vi "User selection GUI.vi"(11 "error in (no error)":errorcluster) -> (8 "OK":bool, 15 "error out":errorcluster)   [LabVIEW 2011]
uses:
  Application Structure/User Control/Super User bool indikator.ctl
  Application Structure/User Control/User Indikator.ctl
  emi Lib/Basic/0 - General/App/Version/Private/_emi_Version Holder.vi
panel:
  in  "User name":string
  in  "Help":bool
  in  "Cancel":bool
  in  "OK btn":bool
  # "Select user name and level"
  # "Tab header s can be changed as wanted\n\nCustom can be used for completly ccutom behavior,\nmust then highjack  an other hidden page, for settings"
  # "Add custom behavior taht cvan not be replicated by a simple cluster with valisdity checking"
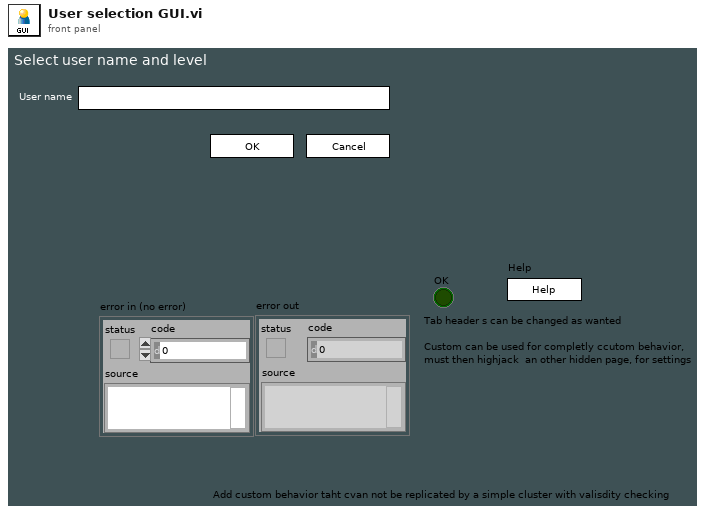
[diagram p1: front panel]
types:
  T1 = enum16{"GET", "SET", "Get from Ini", "Put in Ini"}
  T2 = typedef "User Indikator.ctl" = cluster{"User Name":string, "Super User":T3}
  T3 = typedef "Super User bool indikator.ctl" = bool
  T4 = typedef "emi_Version Info.ctl" = cluster{"Name":string, "Major":i16, "Minor":i16, "Fix":i16, "Build":i32, "Type":enum16{"Alfa", "Beta", "Stable"}, "Dev":bool, "Version Name":string, "Date":timestamp}
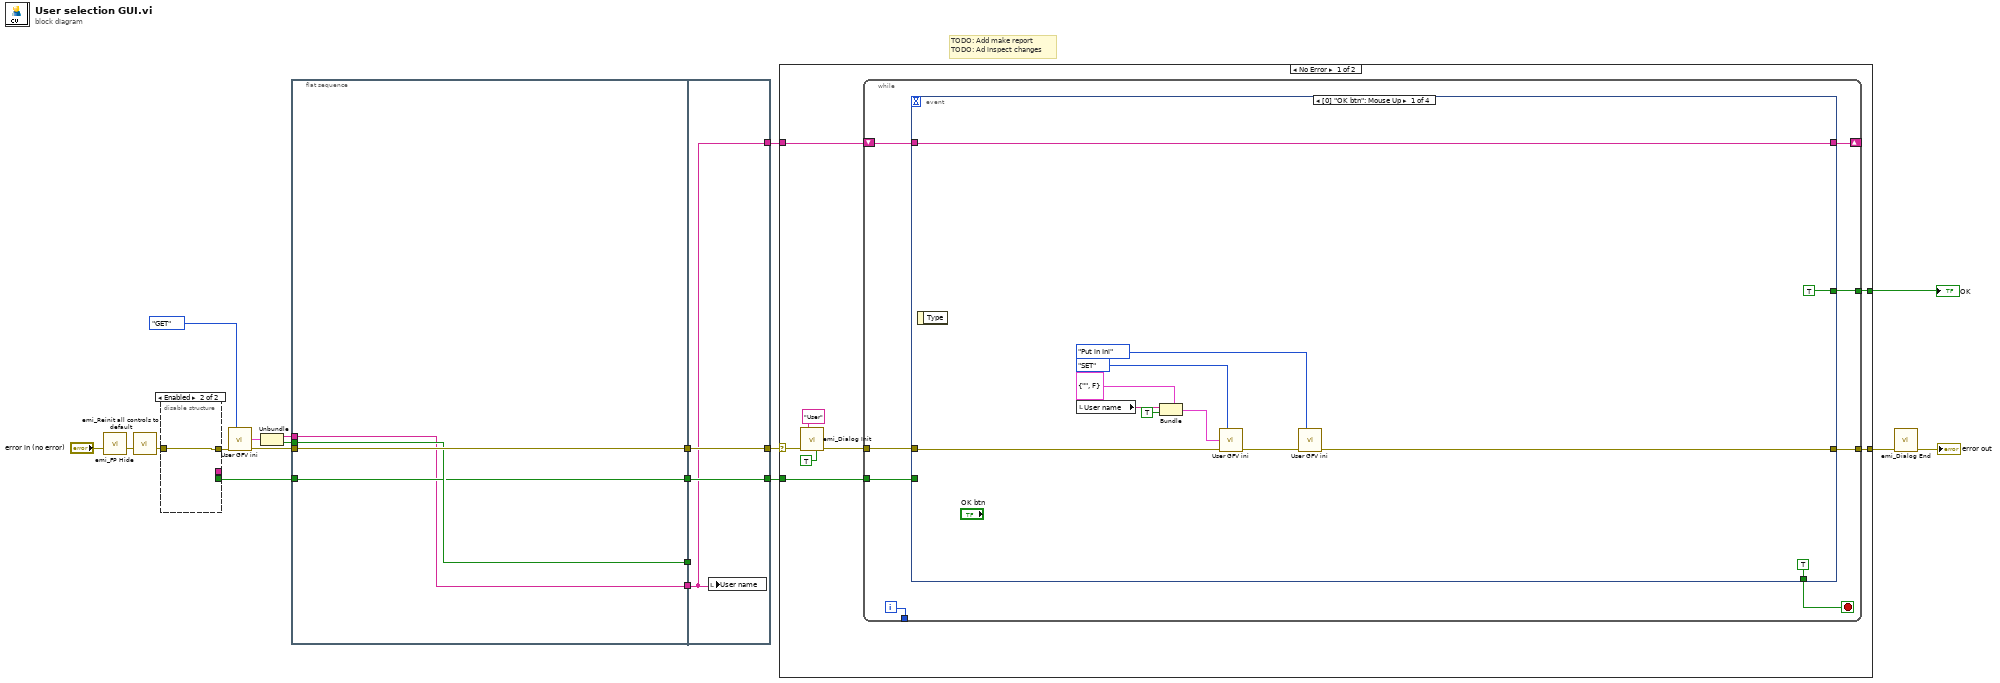
[diagram p0: block diagram]
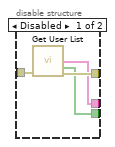
[diagram p2: hidden frame]
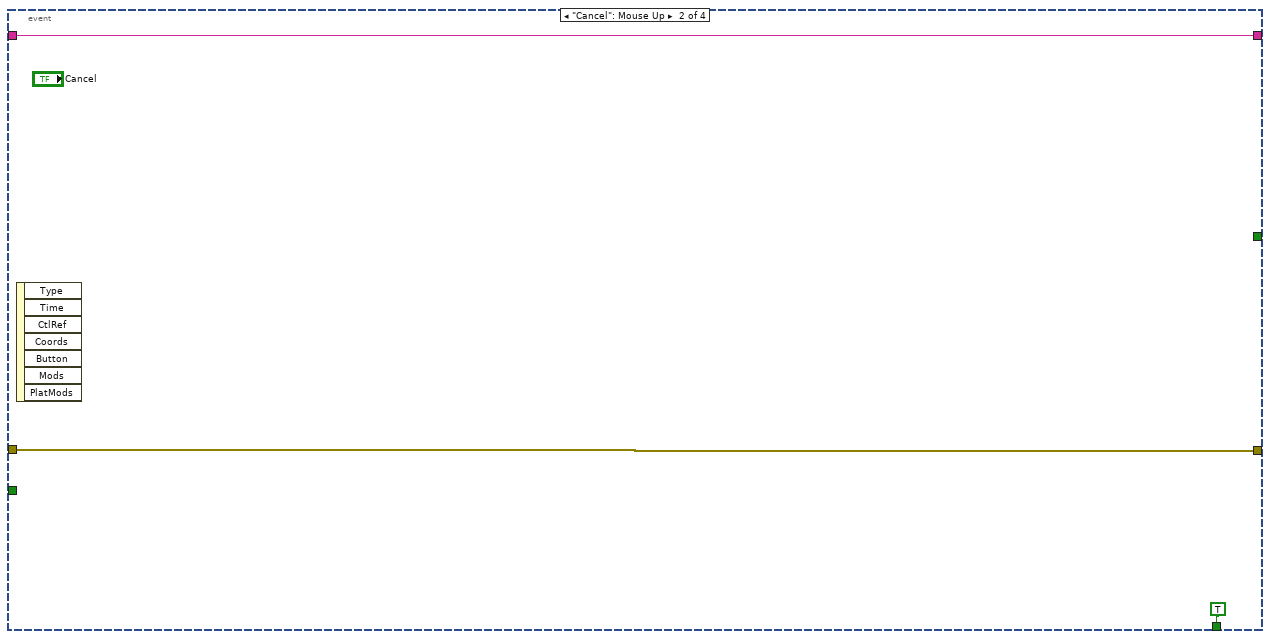
[diagram p3: hidden frame]
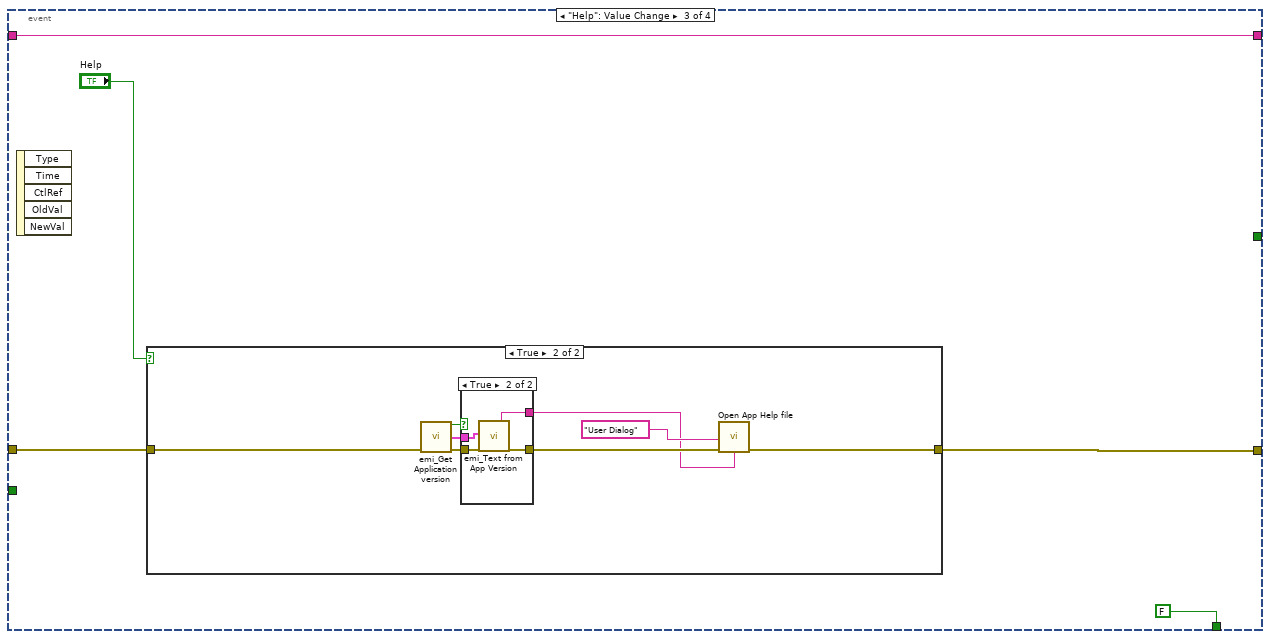
[diagram p4: hidden frame]
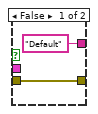
[diagram p6: hidden frame]
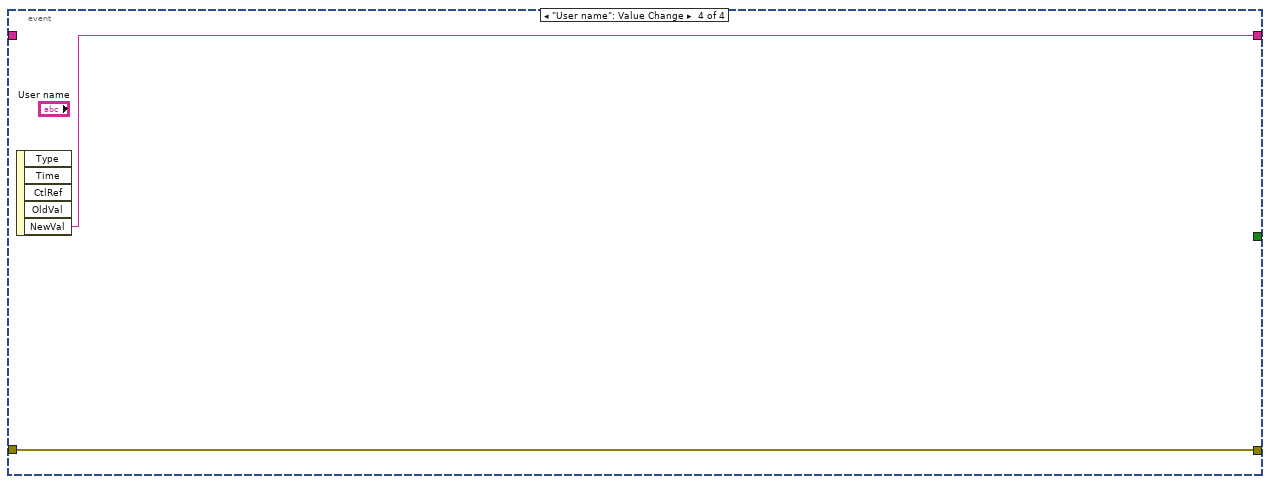
[diagram p7: hidden frame]
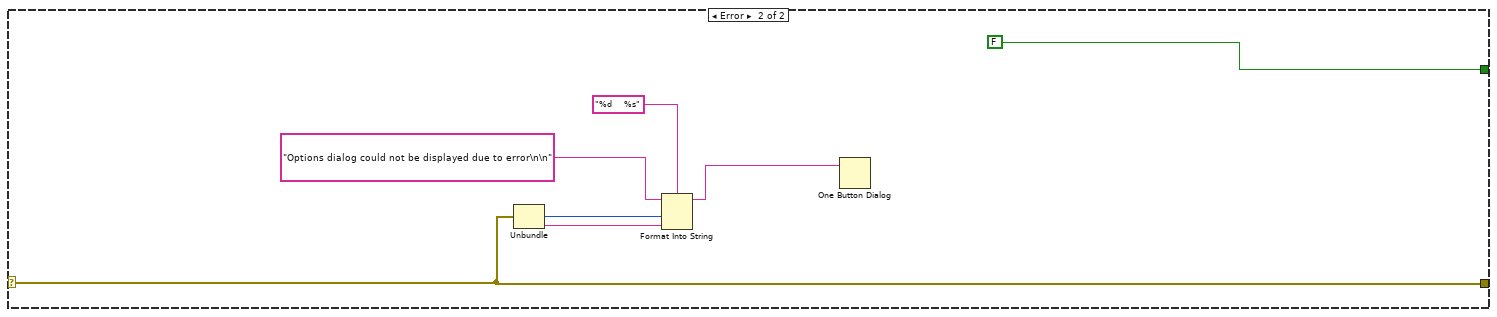
[diagram p8: hidden frame]
diagram:
  # "TODO: Add make report\nTODO: Ad inspect changes"
  n1 = call "emi_FP Hide.vi"("error in (no error)"="error in (no error)") -> ("error out"=w16:errorcluster)  [unwired: 13 in, 1 out]
  n2 = call "emi_Reinit all controls to default.vi"("error in (no error)"=w16) -> ("error out"=w9:errorcluster)  [unwired: 13 in, 1 out]
  n3 = disable-structure shown="Enabled" {
    disable-tunnel: w9 -> [w24 w25]
    disable-tunnel: [w23 w25] -> w8
    disable-tunnel: [w22 _] -> _
    disable-tunnel: [w21 _] -> w7
    frame Disabled {
      n4 = call "Get User List.vi"("error in (no error)"=w24) -> ("Names"=w22:string[], "SU?"=w21:bool[], "error out"=w23:errorcluster)  [unwired: 12 in]
    }
    frame Enabled {
    }
  }
  n5 = call "User GFV ini.vi"("Action(GET)"=T1."GET", "error in (no error)"=w8) -> ("User ID out"=w14:T2, "error out"=w13:errorcluster)  [unwired: 12 in]
  n6 = Unbundle(w14) -> ("User Name"=w10:string, "Super User"=w12:T3)
  n7 = flat-sequence {
    tunnel: w13 -> [w29]
    tunnel: w12 -> [w28]
    tunnel: w10 -> [w26]
    tunnel: w7 -> [w27]
    tunnel: [w29] -> w6
    tunnel: [w26] -> w5
    tunnel: [w28] -> w4
    tunnel: [w27] -> w2
    tunnel: [w32] -> w15
    tunnel: w6 -> [w32]
    tunnel: w5 -> [w30]
    tunnel: w4 -> [_]
    tunnel: [w31] -> w3
    tunnel: w2 -> [w31]
    tunnel: [w30] -> w1
    frame #0 {
    }
    frame #1 {
      n8 = local write "User name"(w30) -> ()
    }
  }
  n9 = case shown="No Error" w15 {
    selector: w15 -> [w35 w91]
    tunnel: [w40 FALSE] -> w19
    tunnel: [w39 w91] -> w18
    tunnel: w3 -> [w34 _]
    tunnel: w1 -> [w33 _]
    frame No Error {
      n10 = call "emi_Dialog Init.vi"("Header String(\"\")"="User" ("Header String(\"\")"), "error in"=w35, "Modal(T)"=TRUE) -> ("error out"=w38:errorcluster)  [unwired: 12 in]
      n11 = while {
        tunnel: [w48] -> _
        tunnel: w38 -> [w46]
        tunnel: [w45] -> w39
        tunnel: [w44] -> w40
        shift-right: [w42] -> _
        shift-left: w33 -> [w43]
        tunnel: w34 -> [w41]
        i -> [w48]
        stop <- w47 stop-if-true
        n12 = event shown="[0] \"OK btn\": Mouse Up" {
          selector: _ -> [_ _ _ _]
          dyn-events: _ -> [_ _ _ _]
          timeout: _ -> [_ _ _ _]
          tunnel: [TRUE TRUE FALSE _] -> w47
          tunnel: w46 -> [w57 w62 w66 w85]
          tunnel: [w51 w62 w67 w85] -> w45
          tunnel: [TRUE _ _ _] -> w44
          tunnel: w43 -> [w59 w61 w64 _]
          tunnel: [w59 w61 w64 w84] -> w42
          tunnel: w41 -> [_ _ _ _]
          event "OK btn": Mouse Up {
            n13 = event-data() -> ()  [unwired: 1 in, 1 out]
            n14 = local read "User name"() -> (w50:string)
            n15 = Bundle(cluster=T2 {"User Name"="", "Super User"=FALSE} ("User ID out"), "User Name"=w50, "Super User"=T3 TRUE) -> (w54:T2)
            n16 = call "User GFV ini.vi"("Action(GET)"=T1."SET", "User ID in"=w54, "error in (no error)"=w57) -> ("error out"=w53:errorcluster)  [unwired: 11 in, 1 out]
            n17 = call "User GFV ini.vi"("Action(GET)"=T1."Put in Ini", "error in (no error)"=w53) -> ("error out"=w51:errorcluster)  [unwired: 12 in, 1 out]
          }
          event "Cancel": Mouse Up {
            n18 = event-data() -> ()  [unwired: 1 in, 7 out]
          }
          event "Help": Value Change {
            n19 = event-data() -> ()  [unwired: 1 in, 5 out]
            n20 = case shown="True" "Help" {
              tunnel: [w69 w70] -> w67
              tunnel: w66 -> [w69 w71]
              frame False {
              }
              frame True {
                n21 = call "emi_Get Application version.vi"("error in (no error)"=w71) -> ("Version has been set"=w75:bool, "Version Info out"=w74:T4, "error out"=w73:errorcluster)  [unwired: 12 in]
                n22 = case shown="True" w75 {
                  tunnel: w73 -> [w79 w83]
                  tunnel: w74 -> [_ w82]
                  tunnel: [w79 w81] -> w77
                  tunnel: ["Default" w80] -> w72
                  frame False {
                  }
                  frame True {
                    n23 = call "emi_Text from App Version.vi"("Version Info"=w82, "error in (no error)"=w83) -> ("Name"=w80:string, "error out"=w81:errorcluster)  [unwired: 8 in, 8 out]
                  }
                }
                n24 = call "Open App Help file.vi"("Help Tag (\"\")"="User Dialog" ("Help Tag (\"\")"), "error In"=w77, "file name(\"App\".chm)"=w72) -> ("error out"=w70:errorcluster)  [unwired: 12 in]
              }
            }
          }
          event "User name": Value Change {
            n25 = event-data() -> ("NewVal"=w84:string)  [unwired: 1 in, 4 out]
          }
        }
      }
    }
    frame Error {
      n26 = Unbundle(w91) -> ("code"=w88:i32, "source"=w87:string)  [unwired: 1 out]
      n27 = Format Into String(format string="%d    %s", initial string="Options dialog could not be displayed due to error\n\n" ("message"), w88, w87) -> (resulting string=w89:string)  [unwired: 1 in, 1 out]
      n28 = One Button Dialog(message=w89) -> ()  [unwired: 1 in, 1 out]
    }
  }
  "OK" <- w19
  n29 = call "emi_Dialog End.vi"("error in"=w18) -> ("error out"=→"error out":errorcluster)  [unwired: 14 in]
